vi "Daten Serialisieren - Statuswerte.vi"(9 "Frame-ID":u32, 10 "Aktuelle Zeit":timestamp, 11 "Messdaten":sgl[](array[numeric])) -> (0 "Frame-ID letzter Wert":u32, 2 "data":T1[](array[typedef])=[{"timestamp"=timestamp(0 s since 1904-01-01), "payload"=[0, 2, 3, 4, 5, 6, 7, 8], "identifier"=2, "type"=0, "extended?"=FALSE, "echo?"=FALSE}, {"timestamp"=timestamp(0 s since 1904-01-01), "payload"=[0, 1, 2, 3, 4, 5, 6, 7], "identifier"=3, "type"=0, "extended?"=FALSE, "echo?"=FALSE}] {"payload" format="%x"; "timestamp" format="%<%.7X\n%x>T"; "type" items=["CAN Data"=0, "CAN Remote"=1, "CAN Bus Error"=2, "CAN 2.0 Data"=8, "CAN FD Data"=16, "CAN FD+BRS Data"=24, "J1939 Data"=192, "Delay"=224, "Log Trigger"=225, "Start Trigger"=226]; "identifier" format="%x"})   [LabVIEW 2020, in "CAN Interface.lvlib"]
uses:
  195161_2023-03-15/cRIO/CAN Interface/CAN Interface.lvlib
  <vilib>/xnet/xnet.llb/XNET Frame Type CAN.ctl
  <vilib>/xnet/xnet.llb/XNET Frame CAN.ctl
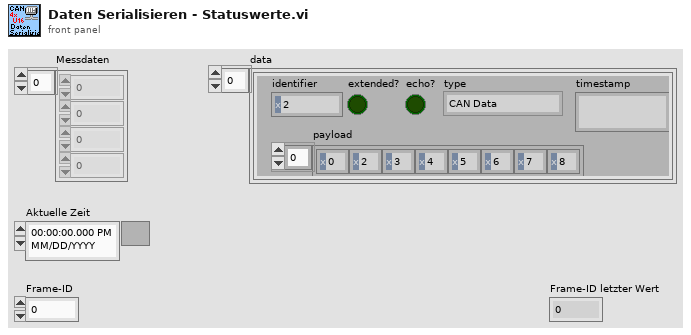
[diagram p1: front panel]
types:
  T1 = typedef "XNET Frame CAN.ctl" = cluster{"timestamp":timestamp, "payload":u8[], "identifier":u32, "type":T2, "extended?":bool, "echo?":bool}
  T2 = typedef "XNET Frame Type CAN.ctl" = u8
  T3 = enum16{"big-endian, network order", "native, host order", "little-endian"}
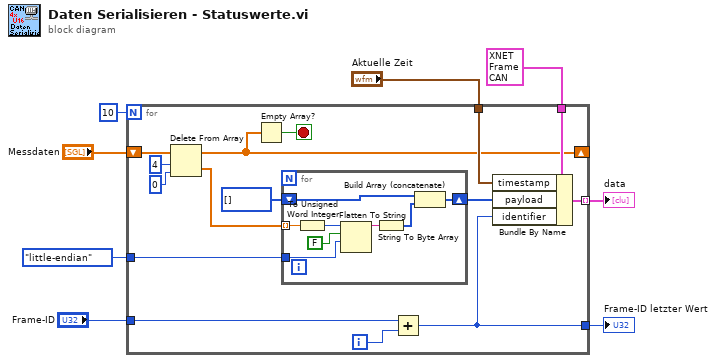
[diagram p0: block diagram]
diagram:
  n1 = for {
    N: 10 -> [_]
    tunnel: T3."little-endian" ("Byte-Reihenfolge (0:Big-Endian, Netzwerkreihenfolge)") -> [w10]
    tunnel: T1 {"timestamp"=timestamp(0 s since 1904-01-01), "payload"=[0, 2, 3, 4, 5, 6, 7, 8], "identifier"=2, "type"=0, "extended?"=FALSE, "echo?"=FALSE} ("CAN frame") -> [w23]
    tunnel: "Frame-ID" -> [w21]
    tunnel: "Aktuelle Zeit" -> [w20]
    tunnel: [w19] -> w4 mode=indexing
    shift-right: [w15] -> _
    shift-left: "Messdaten" -> [w18]
    tunnel: [w9] -> w1
    i -> [w22]
    stop <- w14 stop-if-true
    n2 = Delete From Array(array=w18, length=4 ("Länge"), index=0 ("Index")) -> (deleted portion=w13:sgl[], array with subset deleted=w15:sgl[])
    n3 = Empty Array?(array=w15) -> (empty?=w14:bool)
    n4 = for {
      tunnel: w13 -> [w28] mode=indexing
      shift-right: [w24] -> w11
      shift-left: u8[] [] ("Vorzeichenloses Byte-Array") -> [w25]
      tunnel: w10 -> [w27]
      n5 = To Unsigned Word Integer(number=w28) -> (unsigned 16bit integer=w31:u16)
      n6 = Flatten To String(anything=w31, prepend array or string size? (T)=FALSE ("Array- oder String-Größe voranstellen? (T)"), byte order (0:big-endian, network order)=w27) -> (data string=w30:string)  [unwired: 1 in, 2 out]
      n7 = String To Byte Array(string=w30) -> (unsigned byte array=w26:u8[])
      n8 = Build Array (concatenate)(w25, w26) -> (w24:u8[])
    }
    n9 = Add(x=w21, y=w22) -> (x+y=w9:u32)
    n10 = Bundle By Name(cluster=w23, "timestamp"=w20, "payload"=w11, "identifier"=w9) -> (w19:T1)
  }
  "data" <- w4
  "Frame-ID letzter Wert" <- w1
